vi "Timer Done.vi"(11 "Wait\nTime":dbl) -> (3 "Timer \nDone?":bool)   [LabVIEW 2019]
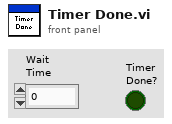
[diagram p1: front panel]
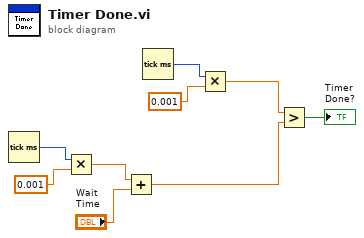
[diagram p0: block diagram]
diagram:
  n1 = Tick Count (ms)() -> (millisecond timer value=w5:u32)
  n2 = Multiply(x=w5, y=0.001) -> (x*y=w4:dbl)
  n3 = Add(x=w4, y="Wait\nTime") -> (x+y=w2:dbl)
  n4 = Tick Count (ms)() -> (millisecond timer value=w8:u32)
  n5 = Multiply(x=w8, y=0.001) -> (x*y=w7:dbl)
  n6 = Greater?(x=w7, y=w2) -> (0:→"Timer \nDone?":bool)
